vi "VI Tree.vi"   [LabVIEW 2012, in "Phidget Distance Sensor.lvlib"]
doc: "${DistanceSensor:VITreeHeader}"
uses:
  <instrlib>/Phidgets/Phidget Distance Sensor/Phidget Distance Sensor.lvlib
  <instrlib>/Phidgets/Phidget Distance Sensor/Public/DistanceSensorStart.vi
  <instrlib>/Phidgets/Phidget Distance Sensor/Public/DistanceSensorOpen.vi
  <instrlib>/Phidgets/Phidget Distance Sensor/Public/DistanceSensorClose.vi
panel:
  # "(c) 2015 Phidgets Inc..  ALL RIGHTS RESERVED."
  # "SEE DIAGRAM\nFOR VI TREE."
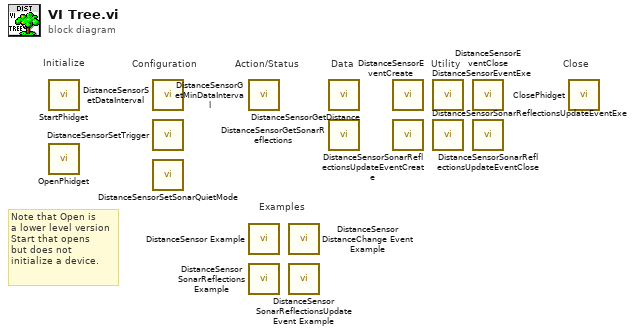
[diagram p0: block diagram]
diagram:
  # "Note that Open is\na lower level version\nStart that opens\nbut does not \ninitialize a device."
  # "Examples"
  # "Configuration"
  # "Utility"
  # "Data"
  # "Action/Status"
  # "Close"
  # "Initialize"
  n1 = call-poly <instrlib>:"StartPhidget.vi"() -> ()  [unwired: 12 in, 4 out]
  n2 = call-poly <instrlib>:"OpenPhidget.vi"() -> ()  [unwired: 8 in, 4 out]
  n3 = call <instrlib>:"DistanceSensorSetDataInterval.vi"() -> ()  [unwired: 9 in, 2 out]
  n4 = call <instrlib>:"DistanceSensorSetTrigger.vi"() -> ()  [unwired: 9 in, 2 out]
  n5 = call <instrlib>:"DistanceSensorSetSonarQuietMode.vi"() -> ()  [unwired: 9 in, 2 out]
  n6 = call <instrlib>:"DistanceSensorGetMinDataInterval.vi"() -> ()  [unwired: 8 in, 3 out]
  n7 = call <instrlib>:"DistanceSensor Example.vi"() -> ()  [unwired: 12 in]
  n8 = call <instrlib>:"DistanceSensor SonarReflections Example.vi"() -> ()  [unwired: 12 in]
  n9 = call <instrlib>:"DistanceSensor DistanceChange Event Example.vi"() -> ()  [unwired: 12 in]
  n10 = call <instrlib>:"DistanceSensor SonarReflectionsUpdate Event Example.vi"() -> ()  [unwired: 12 in]
  n11 = call <instrlib>:"DistanceSensorGetDistance.vi"() -> ()  [unwired: 8 in, 3 out]
  n12 = call <instrlib>:"DistanceSensorGetSonarReflections.vi"() -> ()  [unwired: 11 in, 5 out]
  n13 = call <instrlib>:"DistanceSensorEventCreate.vi"() -> ()  [unwired: 9 in, 3 out]
  n14 = call <instrlib>:"DistanceSensorSonarReflectionsUpdateEventCreate.vi"() -> ()  [unwired: 9 in, 3 out]
  n15 = call <instrlib>:"DistanceSensorEventExe.vi"() -> ()  [unwired: 5 in, 7 out]
  n16 = call <instrlib>:"DistanceSensorSonarReflectionsUpdateEventExe.vi"() -> ()  [unwired: 11 in, 9 out]
  n17 = call <instrlib>:"DistanceSensorEventClose.vi"() -> ()  [unwired: 10 in, 2 out]
  n18 = call <instrlib>:"DistanceSensorSonarReflectionsUpdateEventClose.vi"() -> ()  [unwired: 10 in, 2 out]
  n19 = call-poly <instrlib>:"ClosePhidget.vi"() -> ()  [unwired: 11 in, 1 out]
